vi "Specify Target Info.vi"(11 "target location":T1) -> (0 "skew":dbl, 1 "area":dbl, 2 "offsetAngle V":dbl, 3 "offsetAngle H":dbl, 4 "output":T1)   [LabVIEW 2019]
uses:
  <vilib>/Rock Robotics/Network Tables/NT Read Number.vi
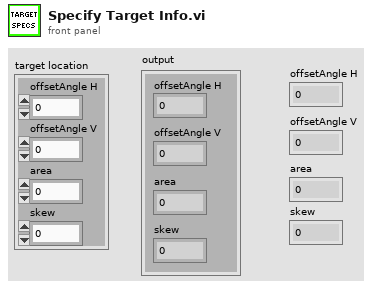
[diagram p1: front panel]
types:
  T1 = cluster{"offsetAngle H":dbl, "offsetAngle V":dbl, "area":dbl, "skew":dbl}
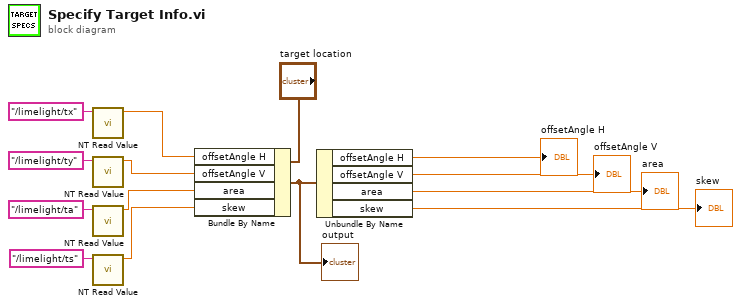
[diagram p0: block diagram]
diagram:
  n1 = call-poly <vilib>:"NT Read Value.vi"("Name"="/limelight/tx") -> ("Numeric"=w7:dbl)  [unwired: 9 in, 1 out]
  n2 = call-poly <vilib>:"NT Read Value.vi"("Name"="/limelight/ty") -> ("Numeric"=w8:dbl)  [unwired: 9 in, 1 out]
  n3 = call-poly <vilib>:"NT Read Value.vi"("Name"="/limelight/ta") -> ("Numeric"=w9:dbl)  [unwired: 9 in, 1 out]
  n4 = call-poly <vilib>:"NT Read Value.vi"("Name"="/limelight/ts") -> ("Numeric"=w10:dbl)  [unwired: 9 in, 1 out]
  n5 = Bundle By Name(cluster="target location", "offsetAngle H"=w7, "offsetAngle V"=w8, "area"=w9, "skew"=w10) -> (w11:T1)
  "output" <- w11
  n6 = Unbundle By Name(w11) -> ("offsetAngle H"=→"offsetAngle H":dbl, "offsetAngle V"=→"offsetAngle V":dbl, "area"=→"area":dbl, "skew"=→"skew":dbl)
